vi "Timer_Core.vi"(8 "error in (no error)":errorcluster caption="错误输入（无错误）", 11 "Timer 输入":refnum<class "Timer.lvclass">) -> (0 "error out":errorcluster caption="错误输出", 3 "Timer 输出":refnum<class "Timer.lvclass">)   [LabVIEW 2019, in "Timer.lvclass"]
uses:
  Timer.lvclass
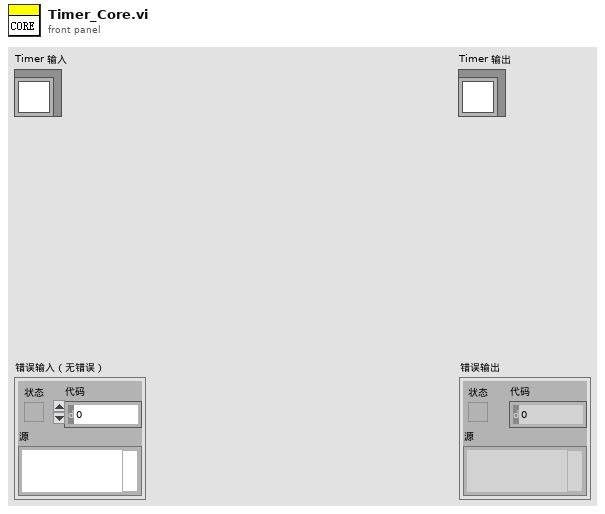
[diagram p1: front panel]
types:
  T1 = typedef "Timer.lvclass/Attribute.ctl" = cluster{"计时？":bool, "计时 (ms)":u32, "core引用":refnum<vi>, "停止通知":refnum<notifier>}
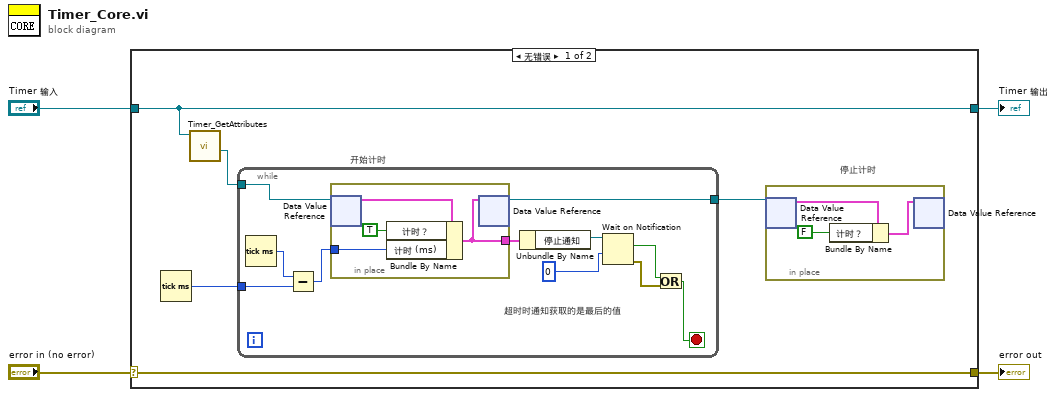
[diagram p0: block diagram]
diagram:
  n1 = case shown="无错误" "error in (no error)" {
    selector: "error in (no error)" -> [w9 w29]
    tunnel: [w9 w29] -> w3
    tunnel: [w7 w28] -> w1
    tunnel: "Timer 输入" -> [w7 w28]
    frame No Error {
      # "停止计时"
      # "开始计时"
      n2 = Tick Count (ms)() -> (millisecond timer value=w8:u32)
      n3 = call "Timer_GetAttributes.vi"("Timer 输入"=w7) -> ("数据值引用"=w6:refnum<data-value>)  [unwired: 7 in, 3 out]
      n4 = while {
        tunnel: w8 -> [w19]
        tunnel: w6 -> [w23]
        tunnel: [w21] -> w5
        stop <- w14 stop-if-true
        # "超时时通知获取的是最后的值"
        n5 = Tick Count (ms)() -> (millisecond timer value=w20:u32)
        n6 = Subtract(x=w20, y=w19) -> (x-y=w22:u32)
        n7 = in-place {
          in-place-border: w22 -> [w25]
          in-place-border: [w24] -> w18
          n8 = in-place-dvr #1(w23) -> (w27:T1)  [unwired: 1 out]
          n9 = Bundle By Name(cluster=w27, "计时？"=TRUE, "计时 (ms)"=w25) -> (w24:T1)
          n10 = in-place-dvr #1(w24) -> (w21:refnum<data-value>)  [unwired: 1 out]
        }
        n11 = Unbundle By Name(w18) -> ("停止通知"=w17:refnum<notifier>)
        n12 = Wait on Notification(notifier=w17, timeout in ms (-1)=0 ("超时毫秒(-1)")) -> (notification=w13:bool, error out=w15:errorcluster)  [unwired: 2 in, 2 out]
        n13 = Or(x=w13, y=w15) -> (x .or. y?=w14:bool)
      }
      n14 = in-place {
        n15 = in-place-dvr #2(w5) -> (w12:T1)  [unwired: 1 out]
        n16 = Bundle By Name(cluster=w12, "计时？"=FALSE) -> (w10:T1)
        n17 = in-place-dvr #2(w10) -> ()  [unwired: 2 out]
      }
    }
    frame Error {
    }
  }
  "error out" <- w3
  "Timer 输出" <- w1
